vi "WriteEprom.vi"() -> ()   [LabVIEW 2017]
uses:
  Traverse/ICNC/ICNC2.lvlib
panel:
  in  "number":i32
  in  "Numeric 3":i32=1
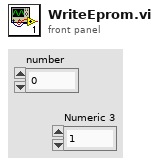
[diagram p1: front panel]
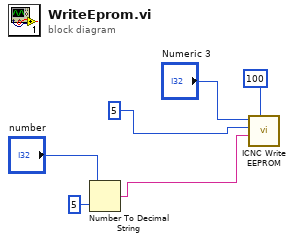
[diagram p0: block diagram]
diagram:
  n1 = Number To Decimal String(number="number", width (-)=i16 5) -> (decimal integer string=w4:string)
  n2 = call <menus>:"ICNC Write EEPROM.vi"("WaitCompletion"=100, "Value"=w4, "Length"=5, "StartAdress"="Numeric 3") -> ()  [unwired: 5 in, 3 out]
